vi "mongo_find_one.vi"(8 "fields":T2, 9 "query":T2, 10 "ns":string, 11 "conn in":T1) -> (0 "error out":errorcluster, 2 "out":T2, 3 "conn out":T1)   [LabVIEW 2013]
uses:
  bson.ctl
  mongo.ctl
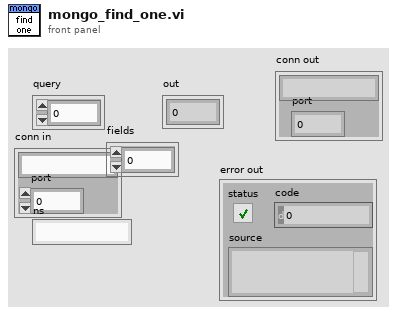
[diagram p1: front panel]
types:
  T1 = typedef "mongo.ctl" = cluster{"host":string, "port":i32}
  T2 = typedef "bson.ctl" = cluster{i32}
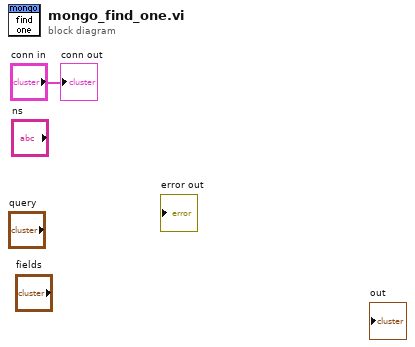
[diagram p0: block diagram]
diagram:
  "conn out" <- "conn in"
